vi "Save Coincidences.vi"   [LabVIEW 2016]
uses:
  Typedefs/Coincidence.ctl
types:
  T1 = typedef "Coincidence.ctl" = cluster{"Primary ID":i8, "Muon hit time":u64, "Secondary ID":i8, "DeltaT":i32}
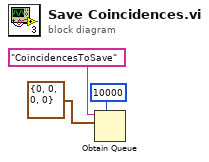
[diagram p0: block diagram]
diagram:
  n1 = Obtain Queue(max queue size (-1, unlimited)=10000, name (unnamed)="CoincidencesToSave", element data type=T1 {"Primary ID"=0, "Muon hit time"=0, "Secondary ID"=0, "DeltaT"=0} ("Coincidence")) -> ()  [unwired: 2 in, 3 out]
